vi "Create RAMP Name.vi"(1 "Numeric 2":dbl, 2 "Numeric 1":dbl, 3 "Prefix":string) -> (0 "concatenated string":string)   [LabVIEW 2013]
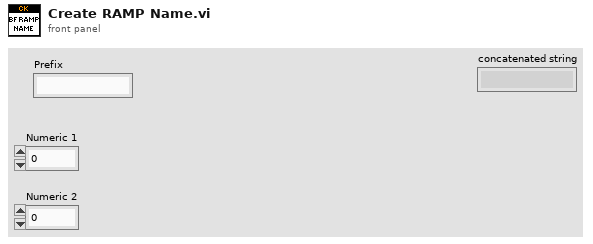
[diagram p1: front panel]
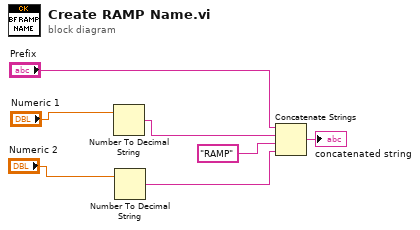
[diagram p0: block diagram]
diagram:
  n1 = Number To Decimal String(number="Numeric 1") -> (decimal integer string=w7:string)  [unwired: 1 in]
  n2 = Number To Decimal String(number="Numeric 2") -> (decimal integer string=w4:string)  [unwired: 1 in]
  n3 = Concatenate Strings("Prefix", w7, "RAMP" ("string"), w4) -> (→"concatenated string":string)
